vi "Execute_SQL_query.vi"() -> ()   [LabVIEW 2024]
uses:
  <vilib>/drjdpowell/SQLite Library/SQL Connection/Open (path).vi
  <vilib>/drjdpowell/SQLite Library/SQL Connection/Open (string).vi
  <vilib>/AdvancedString/Path To Command Line String.vi
  <vilib>/drjdpowell/SQLite Library/SQL Connection/Execute SQL (No results).vi
  <vilib>/drjdpowell/SQLite Library/SQL Connection/Connection.lvclass
  <vilib>/drjdpowell/SQLite Library/SQLite.lvlib
panel:
  out "error out":errorcluster
  in  "SQL query":string
  in  "Path":path
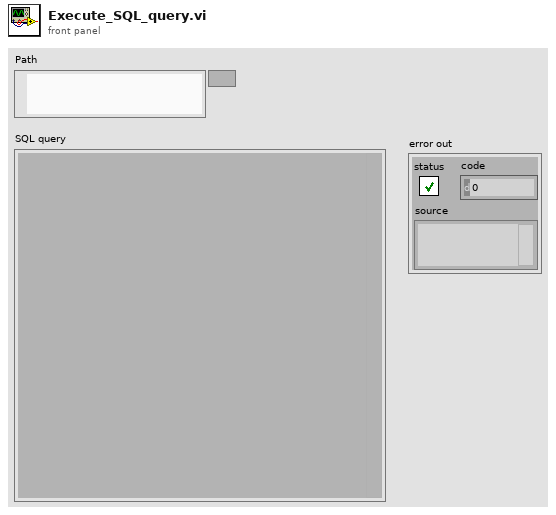
[diagram p1: front panel]
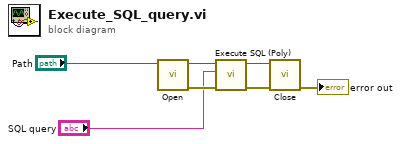
[diagram p0: block diagram]
diagram:
  n1 = call-poly <vilib>:"Open.vi"("db file"="Path") -> ("error out"=w4:errorcluster, "SQLite Connection"=w6:refnum<class "Connection.lvclass">)  [unwired: 9 in]
  n2 = call-poly <vilib>:"Execute SQL (Poly).vi"("error in (no error)"=w4, "SQL"="SQL query", "SQLite Connection in"=w6) -> ("error out"=w3:errorcluster, "SQLite Connection"=w5:refnum<class "Connection.lvclass">)  [unwired: 7 in]
  n3 = call-dynamic "Close.vi"("error in (no error)"=w3, "SQLite Connection in"=w5) -> ("error out"=→"error out":errorcluster)  [unwired: 9 in]
